vi "sutter driver.vi"(0 "VISA resource name":refnum<visa-resource-name>) -> ()   [LabVIEW 2016]
uses:
  <vilib>/Instr/_visa.llb/VISA Configure Serial Port (Instr).vi
panel:
  out "error out":errorcluster
  out "Send Position":dbl[](array[numeric])
  out "Curent Position":dbl[](array[numeric])
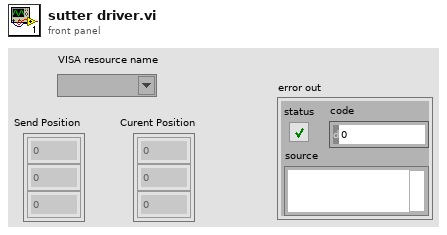
[diagram p1: front panel]
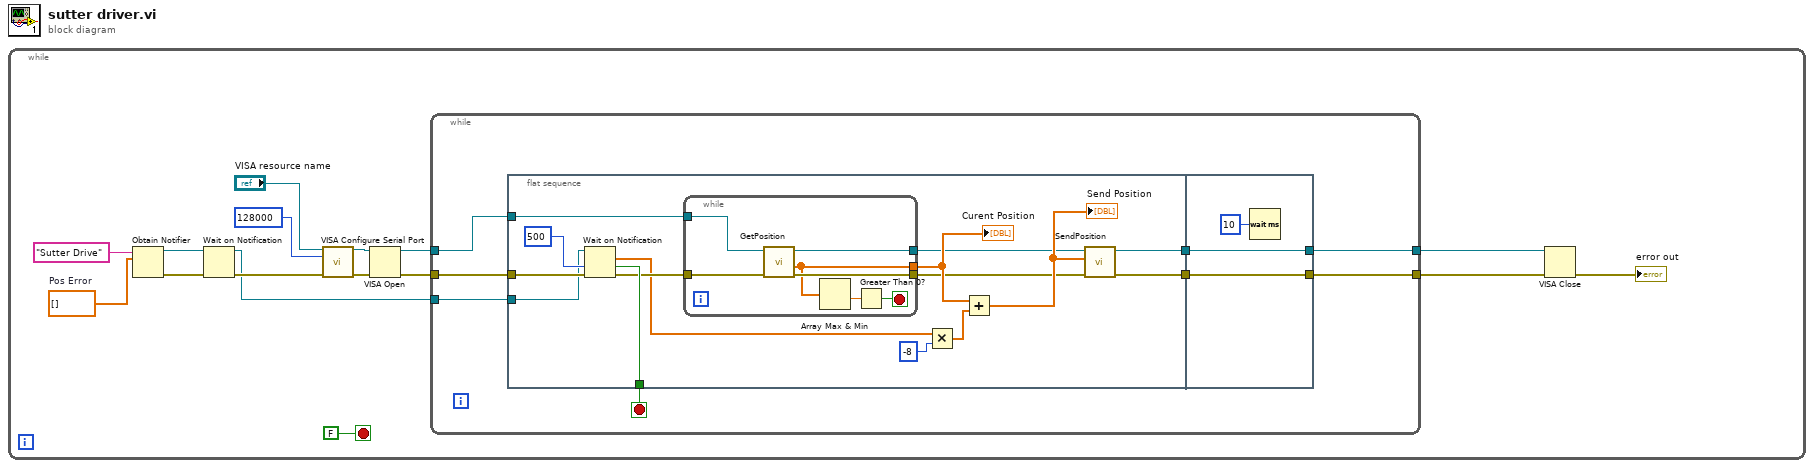
[diagram p0: block diagram]
diagram:
  n1 = while {
    stop <- FALSE stop-if-true
    w5 = dbl[] []  # Pos Error
    n2 = Obtain Notifier(name (unnamed)="Sutter Drive", notification data type=w5) -> (notifier out=w6:refnum<notifier>, error out=w7:errorcluster)  [unwired: 2 in, 1 out]
    n3 = Wait on Notification(notifier=w6, error in (no error)=w7) -> (notifier out=w3:refnum<notifier>, error out=w4:errorcluster)  [unwired: 2 in, 2 out]
    n4 = call-poly "VISA Configure Serial Port"("VISA resource name"="VISA resource name", "baud rate (9600)"=u32 128000, "error in (no error)"=w4) -> ("VISA resource name out"=w14:refnum<visa-resource-name>, "error out"=w13:errorcluster)  [unwired: 11 in]
    n5 = VISA Open(error in (no error)=w13, VISA resource name=w14) -> (VISA resource name=w11:refnum<visa-resource-name>, error out=w10:errorcluster)  [unwired: 3 in]
    n6 = while {
      tunnel: w10 -> [w22]
      tunnel: [w23] -> w8
      tunnel: w11 -> [w21]
      tunnel: [w24] -> w9
      tunnel: w3 -> [w17]
      stop <- w18 stop-if-true
      n7 = flat-sequence {
        tunnel: w22 -> [w29]
        tunnel: w21 -> [w37]
        tunnel: [w39] -> w20
        tunnel: [w38] -> w19
        tunnel: [w30] -> w18
        tunnel: w17 -> [w27]
        tunnel: [w48] -> w23
        tunnel: [w49] -> w24
        tunnel: w20 -> [w49]
        tunnel: w19 -> [w48]
        frame #0 {
          n8 = Wait on Notification(notifier=w27, timeout in ms (-1)=500, error in (no error)=w29) -> (notification=w26:dbl[], timed out?=w30:bool, error out=w28:errorcluster)  [unwired: 1 in, 1 out]
          n9 = while {
            tunnel: [w42] -> w34
            tunnel: w37 -> [w45]
            tunnel: [w44] -> w32
            tunnel: w28 -> [w46]
            tunnel: [w43] -> w31
            stop <- w40 stop-if-true
            n10 = call "GetPosition.vi"("error in"=w46, "VISA resource name in"=w45) -> ("error out"=w43:errorcluster, "Position XYZ"=w42:dbl[], "VISA resource name out"=w44:refnum<visa-resource-name>)  [unwired: 3 in, 1 out]
            n11 = Array Max & Min(array=w42) -> (min value=w41:dbl)  [unwired: 3 out]
            n12 = Greater Than 0?(x=w41) -> (x > 0?=w40:bool)
          }
          "Curent Position" <- w34
          n13 = Multiply(x=w26, y=-8 ("number: 0 to 1")) -> (x*y=w33:dbl[])
          n14 = Add(x=w34, y=w33) -> (x+y=w36:dbl[])
          "Send Position" <- w36
          n15 = call "SendPosition.vi"("error in"=w31, "Motor Position"=w36, "VISA resource In"=w32) -> ("error out"=w38:errorcluster, "VISA resource name out"=w39:refnum<visa-resource-name>)  [unwired: 5 in]
        }
        frame #1 {
          n16 = Wait (ms)(milliseconds to wait=u32 10) -> ()  [unwired: 1 out]
        }
      }
    }
    n17 = VISA Close(VISA resource name=w9, error in (no error)=w8) -> (error out=→"error out":errorcluster)
  }
